vi "Power_spectrum_TF.vi"(5 "Spectrum input array":dbl[](array[numeric]) format="%.2f", 8 "Cluster 1":T2={"Colour"=0, "Inst type"=enum."Pitot-static tube", "Inst name"="Manometer voltage", "Symbol"="U", "Code name"="", "Extra Info"="U", "Inst Array"=enum."PWA", "Index"=0, "Voltage Index"=0, "Extra Titles"=[], "Extra Values"=[], "Eng Values"=[], "Time (ms)"=[], "TT / Voltage"=[], "U"=0.0, "u^2"=0.0, "u^3"=0.0, "u^4"=0.0, "Skew_u"=0.0, "Kurt_u"=0.0, "Mean % Err"=0.0, "% u'/U"=0.0, "X"=0.0, "Y"=0.0, "Z"=0.0, "Spectra"={"First Name"="", "Second Name"="", "X axis name"="", "Y axis name"="", "X array"=[], "Y array"=[]}, "Autocorrelation"={"First Name"="", "Second Name"="", "X axis name"="", "Y axis name"="", "X array"=[], "Y array"=[]}} {"Skew_u" format="%.2f"; "% u'/U" format="%.2f"; "Mean % Err" format="%.2f"; "Kurt_u" format="%.2f"; "u^4" format="%.2f"; "u^3" format="%.2f"; "U" format="%.2f"; "u^2" format="%.2f"}) -> (0 "Spectrum output array":dbl[](array[numeric]) format="%.2f", 2 "XY Graph 2":cluster{dbl[], dbl[]}(graph), 3 "XY Plot Cluster":T1)   [LabVIEW 2011]
uses:
  Controls/Analysis_info_cluster.ctl
  Controls/Inst_type.ctl
  Controls/Instrument_Array.ctl
  Controls/XY_Plot_Cluster.ctl
  Globals/Meas_global.vi
  <vilib>/gmath/NI_Gmath.lvlib
panel:
  in  "method":i32(ring) items=["nearest", "linear", "spline", "cubic Hermite", "Lagrange"]
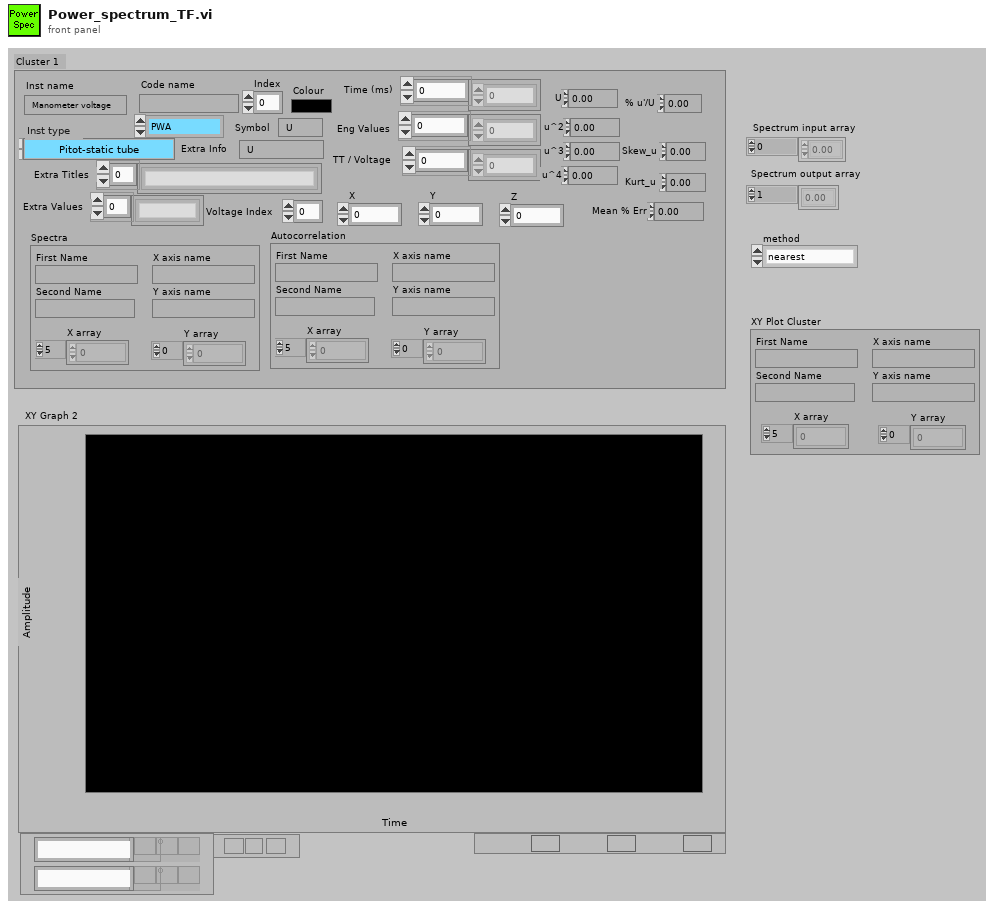
[diagram p1: front panel]
types:
  T1 = typedef "XY_Plot_Cluster.ctl" = cluster{"First Name":string, "Second Name":string, "X axis name":string, "Y axis name":string, "X array":dbl[], "Y array":dbl[]}
  T2 = typedef "Analysis_info_cluster.ctl" = cluster{"Colour":u32, "Inst type":T3, "Inst name":string, "Symbol":string, "Code name":string, "Extra Info":string, "Inst Array":T4, "Index":i32, "Voltage Index":i32, "Extra Titles":string[], "Extra Values":string[], "Eng Values":dbl[], "Time (ms)":dbl[], "TT / Voltage":dbl[], "U":dbl, "u^2":dbl, "u^3":dbl, "u^4":dbl, "Skew_u":dbl, "Kurt_u":dbl, "Mean % Err":dbl, "% u'/U":dbl, "X":dbl, "Y":dbl, "Z":dbl, "Spectra":T1, "Autocorrelation":T1}
  T3 = typedef "Inst_type.ctl" = enum16{"Propeller anemometer", "Raw voltage", "Pressure Transducer", "Pitot-static tube", "Preston tube", "Hot wire", "Cross wire 1", "Cross wire 2", "Generic Linear", "Generic Polynomial", "Generic BackPoly", "Fast FID", "Thermocouple", "Cold wire", "Pulsed Wire", "LDA Vel", "LDA Tran time", "LDA Arr time"}
  T4 = typedef "Instrument_Array.ctl" = enum16{"PWA", "LDA", "Analogue"}
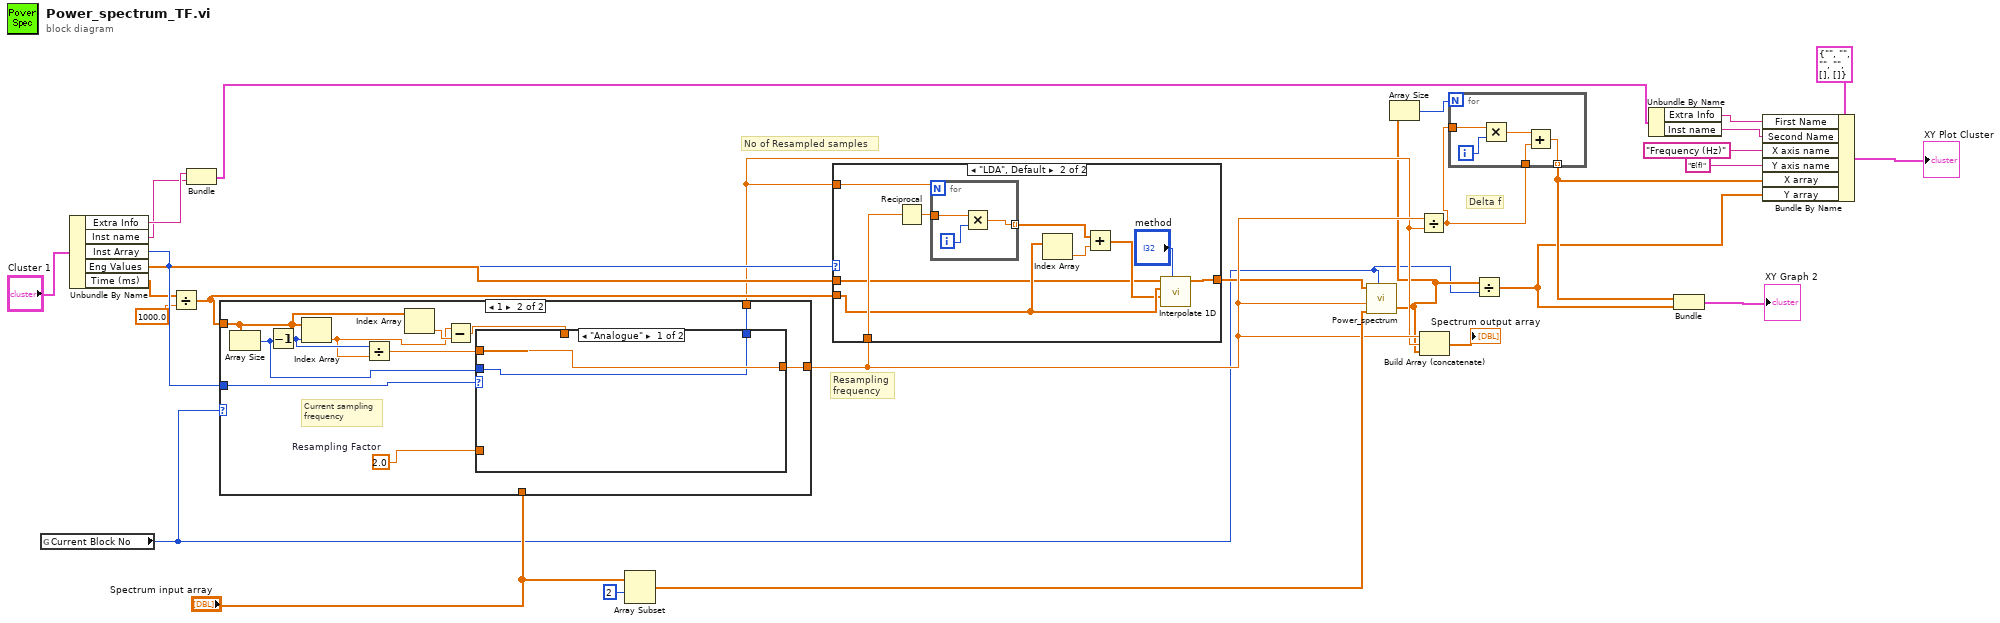
[diagram p0: block diagram]
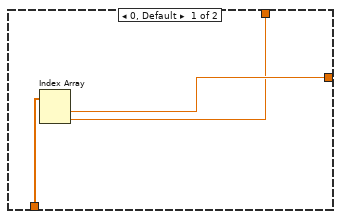
[diagram p2: hidden frame]
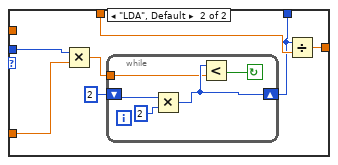
[diagram p3: hidden frame]
diagram:
  # "No of Resampled samples"
  # "Resampling\nfrequency"
  # "Delta f"
  n1 = global read "Meas_global.vi" "Current Block No"() -> (w2:i32)
  n2 = Unbundle By Name("Cluster 1") -> ("Extra Info"=w14:string, "Inst name"=w12:string, "Inst Array"=w23:T4, "Eng Values"=w28:dbl[], "Time (ms)"=w20:dbl[])
  n3 = Divide(x=w20, y=1000.0) -> (x/y=w19:dbl[])
  n4 = Bundle("Extra Info"=w14, "Inst name"=w12) -> (w13:cluster{"Extra Info":string, "Inst name":string})  [unwired: 1 in]
  n5 = case shown="1" w2 {
    tunnel: w19 -> [_ w36]
    tunnel: [w31 w41] -> w22
    tunnel: "Spectrum input array" -> [w32 _]
    tunnel: w23 -> [_ w42]
    tunnel: [w30 w39] -> w16
    frame 0, Default {
      n6 = Index Array(array=w32) -> (element #1=w31:dbl, element #2=w30:dbl)  [unwired: 2 in]
    }
    frame 1 {
      w37 = 2.0  # Resampling Factor
      # "Current sampling\nfrequency"
      n7 = Array Size(array=w36) -> (size(s)=w38:i32)
      n8 = Decrement(x=w38) -> (x-1=w40:i32)
      n9 = Index Array(array=w36, index=w40) -> (element=w33:dbl)
      n10 = Divide(x=w40, y=w33) -> (x/y=w43:dbl)
      n11 = Index Array(array=w36) -> (element=w35:dbl)  [unwired: 1 in]
      n12 = Subtract(x=w33, y=w35) -> (x-y=w34:dbl)
      n13 = case shown="\"Analogue\"" w42 {
        tunnel: w43 -> [w45 _]
        tunnel: w34 -> [_ w52]
        tunnel: [w45 w51] -> w41
        tunnel: w38 -> [w44 w49]
        tunnel: [w44 w48] -> w39
        tunnel: w37 -> [_ w47]
        frame "Analogue" {
        }
        frame "LDA", Default {
          n14 = Multiply(x=w49, y=w47) -> (x*y=w50:dbl)
          n15 = while {
            shift-right: [w55] -> w48
            shift-left: 2 -> [w57]
            tunnel: w50 -> [w53]
            stop <- w54 continue-if-true
            n16 = Multiply(x=w57, y=2) -> (x*y=w55:i32)
            n17 = Less?(x=w55, y=w53) -> (x < y?=w54:bool)
          }
          n18 = Divide(x=w48, y=w52) -> (x/y=w51:dbl)
        }
      }
    }
  }
  n19 = Array Subset(array="Spectrum input array", index=2) -> (w25:dbl[])  [unwired: 1 in]
  n20 = case shown="\"LDA\", Default" w23 {
    tunnel: w28 -> [w58 w59]
    tunnel: w19 -> [_ w63]
    tunnel: [w58 w67] -> w5
    tunnel: w16 -> [_ w66]
    tunnel: w22 -> [_ w64]
    frame "Analogue" {
    }
    frame "LDA", Default {
      n21 = Reciprocal(x=w64) -> (1/x=w65:dbl)
      n22 = for {
        N: w66 -> [_]
        tunnel: w65 -> [w71]
        tunnel: [w69] -> w61 mode=indexing
        i -> [w70]
        n23 = Multiply(x=w71, y=w70) -> (x*y=w69:dbl)
      }
      n24 = Index Array(array=w63) -> (element=w62:dbl)  [unwired: 1 in]
      n25 = Add(x=w61, y=w62) -> (x+y=w60:dbl[])
      n26 = call <vilib>:"Interpolate 1D.vi"("method"="method", "xi"=w60, "X"=w63, "Y"=w59) -> ("yi"=w67:dbl[])  [unwired: 2 in, 5 out]
    }
  }
  n27 = call "Power_spectrum.vi"("U"=w5, "Sampling frequency"=w22, "Spectrum input array"=w25, "Block No"=w2) -> ("Spectrum output array"=w3:dbl[])  [unwired: 2 in]
  n28 = Array Size(array=w3) -> (size(s)=w17:i32)
  n29 = Divide(x=w22, y=w16) -> (x/y=w18:dbl)
  n30 = Build Array (concatenate)(w22, w16, w3) -> (→"Spectrum output array":dbl[])
  n31 = for {
    N: w17 -> [_]
    tunnel: w18 -> [w76]
    tunnel: w18 -> [w73]
    tunnel: [w72] -> w4 mode=indexing
    i -> [w75]
    n32 = Multiply(x=w76, y=w75) -> (x*y=w74:dbl)
    n33 = Add(x=w74, y=w73) -> (x+y=w72:dbl)
  }
  n34 = Divide(x=w3, y=w2) -> (x/y=w1:dbl[])
  n35 = Unbundle By Name(w13) -> ("Extra Info"=w10:string, "Inst name"=w9:string)
  n36 = Bundle(w4, w1) -> (→"XY Graph 2":cluster{dbl[], dbl[]})  [unwired: 1 in]
  n37 = Bundle By Name(cluster=T1 {"First Name"="", "Second Name"="", "X axis name"="", "Y axis name"="", "X array"=[], "Y array"=[]} ("output cluster"), "First Name"=w10, "Second Name"=w9, "X axis name"="Frequency (Hz)", "Y axis name"="E(f)", "X array"=w4, "Y array"=w1) -> (→"XY Plot Cluster":T1)
